vi "MFC-2000 Test Panel.vi"() -> ()   [LabVIEW 2020]
uses:
  <vilib>/Instr/_visa.llb/VISA Configure Serial Port (Instr).vi
panel:
  out "trimmed string":string
  out "Cmd Success":bool
  out "Connected":bool
  out "Waiting for Reply":bool
  out "Last Error":errorcluster
  out "Command History":string
  out "Reply":string
  in  "Command":string
  in  "Quit":bool
  in  "COM Port":refnum<visa-resource-name>="COM4"
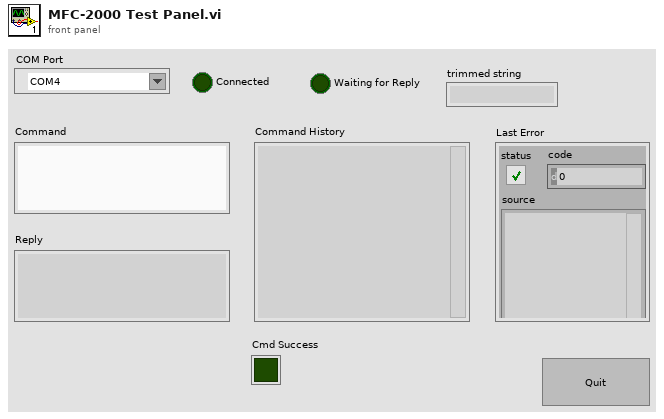
[diagram p1: front panel]
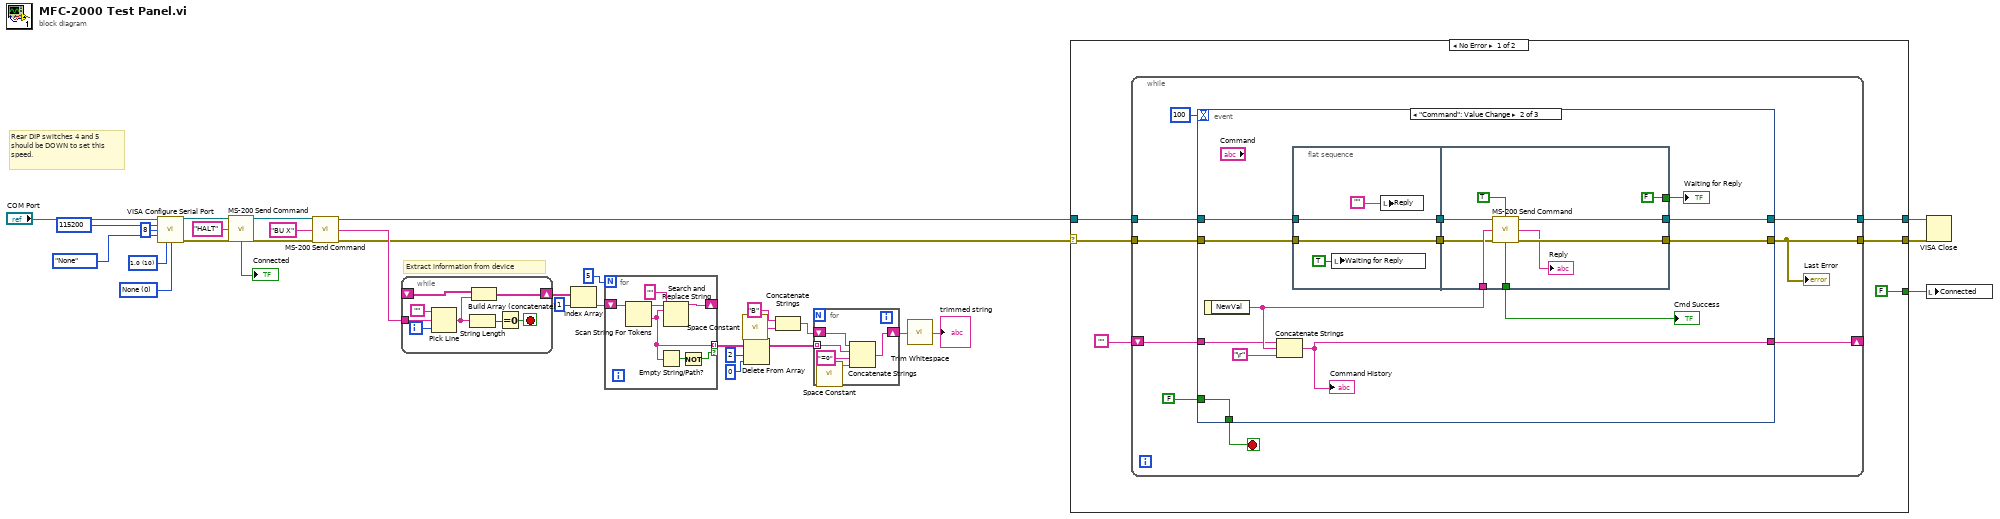
[diagram p0: block diagram]
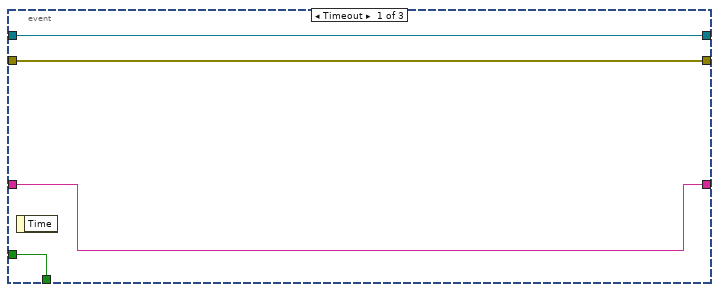
[diagram p2: hidden frame]
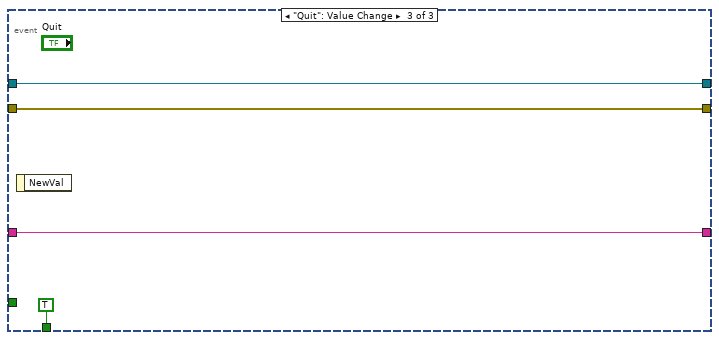
[diagram p3: hidden frame]
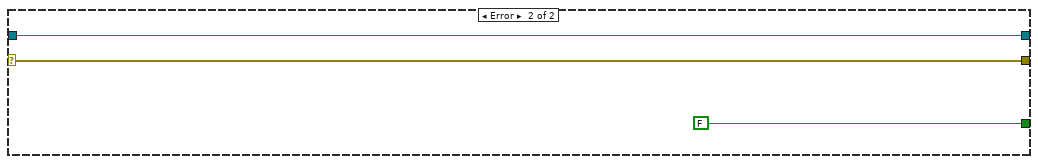
[diagram p4: hidden frame]
diagram:
  w26 = u16 0 items=["None", "XON/XOFF", "RTS/CTS", "XON/XOFF & RTS/CTS", "DTR/DSR", "XON/XOFF & DTR/DSR"] ("flow control (0:none)")
  w29 = u16 10 items=["1.0"=10, "1.5"=15, "2.0"=20] ("stop bits (10: 1 bit)")
  # "Extract information from device"
  # "Rear DIP switches 4 and 5 should be DOWN to set this speed."
  n1 = call-poly "VISA Configure Serial Port"("VISA resource name"="COM Port", "baud rate (9600)"=u32 115200, "data bits (8)"=u16 8, "parity (0:none)"=enum16{"None", "Odd", "Even", "Mark", "Space"}."None", "stop bits (10: 1 bit)"=w29, "flow control (0:none)"=w26) -> ("VISA resource name out"=w5:refnum<visa-resource-name>, "error out"=w6:errorcluster)  [unwired: 8 in]
  n2 = call "MS-200 Send Command.vi"("VISA Ref"=w5, "Command"="HALT", "Error In"=w6) -> ("VISA Ref Dup"=w4:refnum<visa-resource-name>, "Cmd Success"=→"Connected":bool, "Error Out"=w3:errorcluster)  [unwired: 9 in, 1 out]
  n3 = call "MS-200 Send Command.vi"("VISA Ref"=w4, "Command"="BU X", "Error In"=w3) -> ("VISA Ref Dup"=w22:refnum<visa-resource-name>, "Reply"=w21:string, "Error Out"=w20:errorcluster)  [unwired: 9 in, 1 out]
  n4 = while {
    tunnel: w21 -> [w40]
    shift-right: [w38] -> w19
    shift-left: _ -> [w37]
    i -> [w33]
    stop <- w34 stop-if-true
    n5 = Pick Line(string ("")="", multi-line string=w40, line index=w33) -> (output string=w35:string)
    n6 = String Length(string=w35) -> (length=w36:i32)
    n7 = Build Array (concatenate)(w37, w35) -> (w38:string[])
    n8 = Equal To 0?(x=w36) -> (x = 0?=w34:bool)
  }
  n9 = Index Array(array=w19, index=1) -> (element=w16:string)
  n10 = for {
    N: 5 -> [_]
    tunnel: [w43] -> w15 mode=indexing if=w41
    shift-right: [w44] -> _
    shift-left: w16 -> [w47]
    n11 = Scan String For Tokens(9:w47) -> (1:w43:string, 3:w46:string)  [unwired: 5 in, 2 out]
    n12 = Empty String/Path?(string/path=w43) -> (empty?=w42:bool)
    n13 = Search and Replace String(input string=w46, search string=w43, replace string="" ("replace string (\"\")")) -> (result string=w44:string)  [unwired: 5 in, 3 out]
    n14 = Not(x=w42) -> (.not. x?=w41:bool)
  }
  n15 = call <vilib>:"Space Constant.vi"() -> ("String"=w11:string)
  n16 = Delete From Array(array=w15, length=2, index=0) -> (array with subset deleted=w10:string[])  [unwired: 1 out]
  n17 = Concatenate Strings("B", w11) -> (w9:string)
  n18 = for {
    tunnel: w10 -> [w52] mode=indexing
    shift-right: [w50] -> w8
    shift-left: w9 -> [w49]
    n19 = call <vilib>:"Space Constant.vi"() -> ("String"=w48:string)
    n20 = Concatenate Strings(w49, w52, "=0" ("string"), w48) -> (w50:string)
  }
  n21 = call <vilib>:"Trim Whitespace.vi"("string"=w8) -> ("trimmed string"=→"trimmed string":string)  [unwired: 1 in]
  n22 = case shown="No Error" w20 {
    selector: w20 -> [w57 w103]
    tunnel: w22 -> [w58 w104]
    tunnel: [w56 w104] -> w32
    tunnel: [w55 w103] -> w31
    tunnel: [FALSE FALSE] -> w30
    frame No Error {
      n23 = while {
        tunnel: w58 -> [w65]
        tunnel: w57 -> [w64]
        tunnel: [w63] -> w56
        tunnel: [w60] -> w55
        shift-right: [w61] -> _
        shift-left: "" -> [w62]
        stop <- w66 stop-if-true
        n24 = event shown="[1] \"Command\": Value Change" {
          selector: _ -> [_ _ _]
          dyn-events: _ -> [_ _ _]
          timeout: 100 -> [_ _ _]
          tunnel: FALSE -> [w71 w84 _]
          tunnel: [w71 w84 TRUE] -> w66
          tunnel: w65 -> [w69 w83 w101]
          tunnel: w64 -> [w68 w82 w100]
          tunnel: [w69 w78 w101] -> w63
          tunnel: [w68 w79 w100] -> w60
          tunnel: w62 -> [w70 w75 w98]
          tunnel: [w70 w74 w98] -> w61
          event Timeout {
            n25 = event-data() -> ()  [unwired: 1 in, 1 out]
          }
          event "Command": Value Change {
            n26 = event-data() -> ("NewVal"=w77:string)  [unwired: 1 in]
            n27 = Concatenate Strings(w75, w77, "\r") -> (w74:string)
            "Command History" <- w74
            n28 = flat-sequence {
              tunnel: w82 -> [w87]
              tunnel: w83 -> [w88]
              tunnel: [w88] -> w81
              tunnel: [w87] -> w80
              tunnel: w77 -> [w96]
              tunnel: w81 -> [w97]
              tunnel: w80 -> [w95]
              tunnel: [w94] -> w79
              tunnel: [w93] -> w78
              tunnel: [FALSE] -> w73
              tunnel: [w90] -> w72
              frame #0 {
                n29 = local write "Waiting for Reply"(TRUE ("Waiting for Cmd")) -> ()
                n30 = local write "Reply"("") -> ()
              }
              frame #1 {
                n31 = call "MS-200 Send Command.vi"("VISA Ref"=w97, "Wait for Reply (T)"=TRUE, "Command"=w96, "Error In"=w95) -> ("VISA Ref Dup"=w93:refnum<visa-resource-name>, "Reply"=→"Reply":string, "Cmd Success"=w90:bool, "Error Out"=w94:errorcluster)  [unwired: 8 in]
              }
            }
            "Waiting for Reply" <- w73
            "Cmd Success" <- w72
          }
          event "Quit": Value Change {
            n32 = event-data() -> ()  [unwired: 1 in, 1 out]
          }
        }
        "Last Error" <- w60
      }
    }
    frame Error {
    }
  }
  n33 = VISA Close(VISA resource name=w32, error in (no error)=w31) -> ()  [unwired: 1 out]
  n34 = local write "Connected"(w30) -> ()
